vi "construct.vi"(6 "cushion_model":T1 items=["Model 1", "Model 2"], 8 "error in (no error)":errorcluster, 9 "cost":dbl, 10 "id":u32) -> (0 "error out":errorcluster, 3 "IChair.lvclass":refnum<class "IChair.lvclass">)   [LabVIEW 2021]
uses:
  IChair.lvclass
  CushionModel.ctl
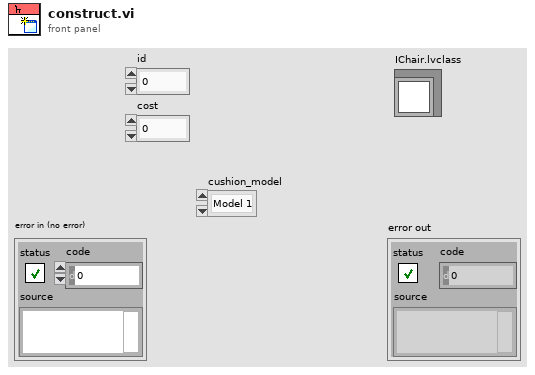
[diagram p1: front panel]
types:
  T1 = typedef "IChair.lvclass/CushionModel.ctl" = u16
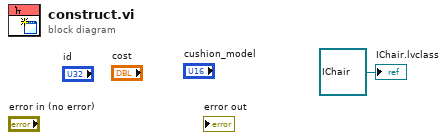
[diagram p0: block diagram]
diagram:
  "IChair.lvclass" <- refnum<class "IChair.lvclass"> refnum ("IChair.lvclass")
